vi "Linear Line.vi"() -> ()   [LabVIEW 2017]
doc: "A linear line is drawn between two points. Input the first point into (x0, x0) and the next point into (x1, y1)."
panel:
  out "XY Graph":cluster{dbl[], dbl[]}(graph)
  out "Y":dbl[](array[numeric])
  out "X":dbl[](array[numeric])
  in  "y0":i32
  in  "y1":i32
  in  "x0":i32
  in  "x1":i32
  # "The linear drawn by this VI uses Digital Differential Analyzer (DDA) algorithm."
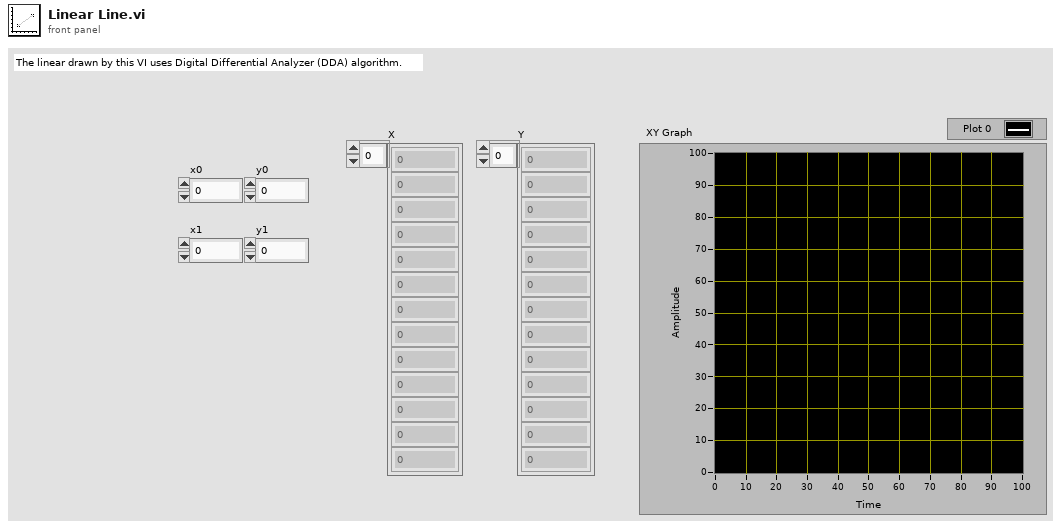
[diagram p1: front panel]
types:
  T1 = enum16{"Full", "Half", "Quarter", "Eighth", "Sixteenth"}
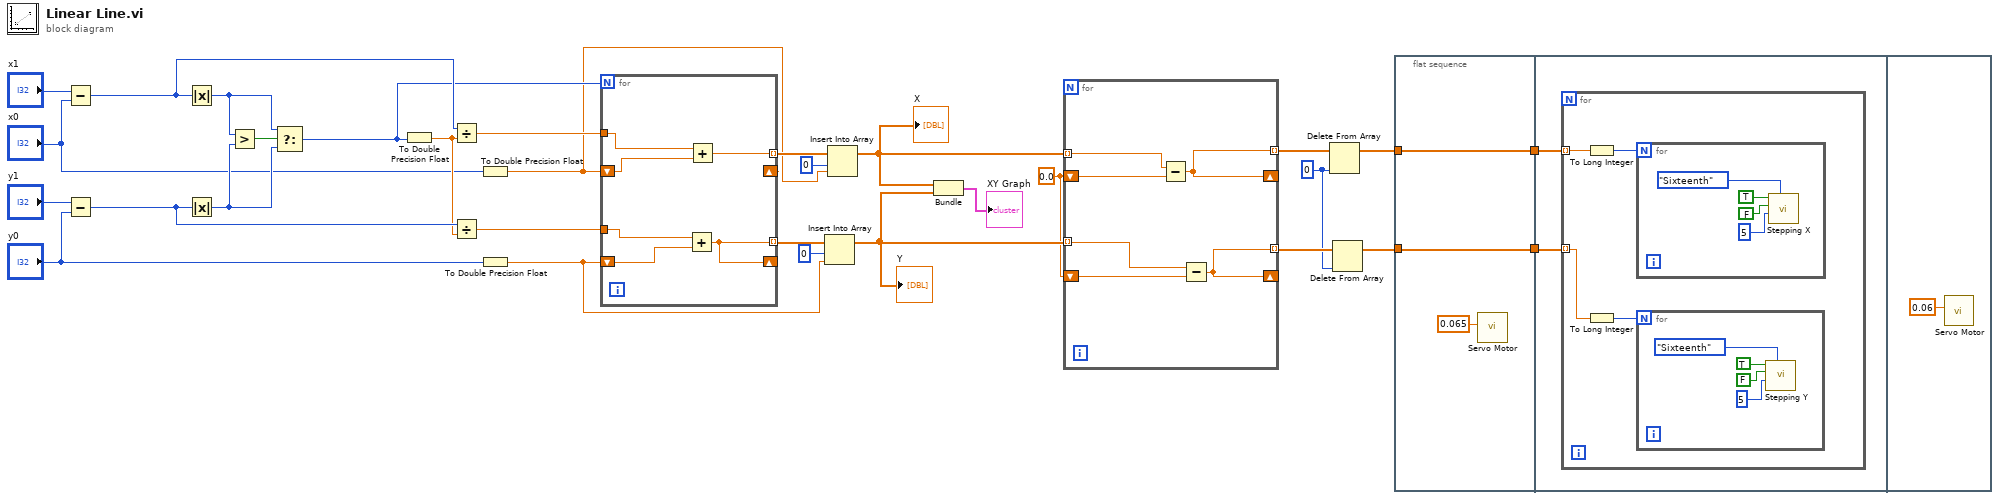
[diagram p0: block diagram]
diagram:
  w5 = 0 ("index")
  w8 = 0.0
  n1 = Subtract(x="x1", y="x0") -> (x-y=w25:i32)
  n2 = Subtract(x="y1", y="y0") -> (x-y=w24:i32)
  n3 = Absolute Value(x=w25) -> (abs(x)=w27:i32)
  n4 = Absolute Value(x=w24) -> (abs(x)=w26:i32)
  n5 = Greater?(x=w27, y=w26) -> (0:w28:bool)
  n6 = Select(t=w27, s=w28, f=w26) -> (s? t:f=w22:i32)
  n7 = To Double Precision Float(number=w22) -> (double precision float=w23:dbl)
  n8 = Divide(x=w25, y=w23) -> (x/y=w21:dbl)
  n9 = Divide(x=w24, y=w23) -> (x/y=w20:dbl)
  n10 = To Double Precision Float(number="x0") -> (double precision float=w15:dbl)
  n11 = To Double Precision Float(number="y0") -> (double precision float=w12:dbl)
  n12 = for {
    N: w22 -> [_]
    tunnel: w21 -> [w36]
    tunnel: w20 -> [w33]
    shift-right: [w34] -> _
    shift-left: w15 -> [w35]
    shift-right: [w31] -> _
    shift-left: w12 -> [w32]
    tunnel: [w34] -> w16 mode=indexing
    tunnel: [w31] -> w14 mode=indexing
    n13 = Add(x=w33, y=w32) -> (x+y=w31:dbl)
    n14 = Add(x=w36, y=w35) -> (x+y=w34:dbl)
  }
  n15 = Insert Into Array(array=w14, index=0, new element=w12) -> (w9:dbl[])
  "Y" <- w9
  n16 = Insert Into Array(array=w16, index=0, new element=w15) -> (w10:dbl[])
  "X" <- w10
  n17 = Bundle(w10, w9) -> (→"XY Graph":cluster{dbl[], dbl[]})  [unwired: 1 in]
  n18 = for {
    shift-right: [w38] -> _
    shift-left: w8 -> [w39]
    shift-right: [w37] -> _
    shift-left: w8 -> [w41]
    tunnel: w10 -> [w42] mode=indexing
    tunnel: w9 -> [w40] mode=indexing
    tunnel: [w38] -> w7 mode=indexing
    tunnel: [w37] -> w6 mode=indexing
    n19 = Subtract(x=w42, y=w39) -> (x-y=w38:dbl)
    n20 = Subtract(x=w40, y=w41) -> (x-y=w37:dbl)
  }
  n21 = Delete From Array(array=w7, index=w5) -> (array with subset deleted=w4:dbl[])  [unwired: 1 in, 1 out]
  n22 = Delete From Array(array=w6, index=w5) -> (array with subset deleted=w3:dbl[])  [unwired: 1 in, 1 out]
  n23 = flat-sequence {
    tunnel: w3 -> [w44]
    tunnel: w4 -> [w45]
    tunnel: [w45] -> w2
    tunnel: [w44] -> w1
    tunnel: w2 -> [w47]
    tunnel: w1 -> [w46]
    frame #0 {
      n24 = call "Servo Motor.vi"("Duty Cycle"=0.065) -> ()  [unwired: 9 in, 2 out]
    }
    frame #1 {
      n25 = for {
        tunnel: w47 -> [w51] mode=indexing
        tunnel: w46 -> [w50] mode=indexing
        n26 = To Long Integer(number=w51) -> (32bit integer=w49:i32)
        n27 = To Long Integer(number=w50) -> (32bit integer=w48:i32)
        n28 = for {
          N: w49 -> [_]
          n29 = call "Stepping X.vi"("Microstep size"=T1."Sixteenth", "Speed"=u32 5, "Direction"=FALSE, "Enable"=TRUE) -> ()  [unwired: 7 in, 1 out]
        }
        n30 = for {
          N: w48 -> [_]
          n31 = call "Stepping Y.vi"("Microstep size"=T1."Sixteenth", "Speed"=u32 5, "Direction"=FALSE, "Enable"=TRUE) -> ()  [unwired: 7 in, 1 out]
        }
      }
    }
    frame #2 {
      n32 = call "Servo Motor.vi"("Duty Cycle"=0.06) -> ()  [unwired: 9 in, 2 out]
    }
  }
